vi "OA Get Mode Acq Params.vi"(8 "error in (no error)":errorcluster, 10 "pcListOfParams":string, 11 "pcModeName":string) -> (0 "error out":errorcluster, 2 "pcListOfParams out":string, 3 "function return":u32)   [LabVIEW 2014, in "atmcd32d.lvlib"]
doc: "unsigned int WINAPI OA_GetModeAcqParams(const char * const pcModeName, char * const pcListOfParams);"
uses:
  atmcd32d.lvlib
  atmcd32d.dll
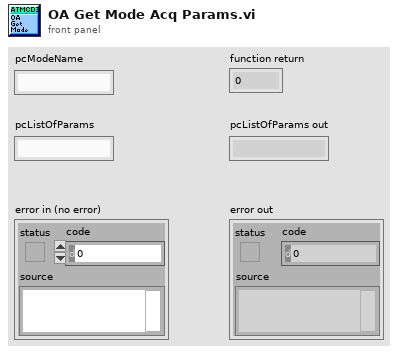
[diagram p1: front panel]
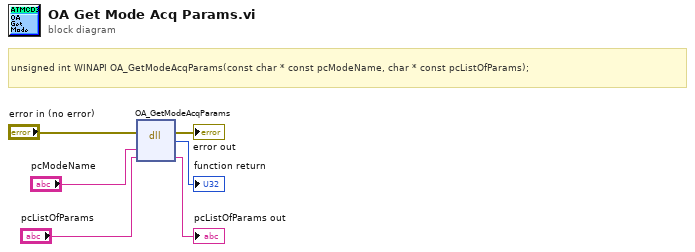
[diagram p0: block diagram]
diagram:
  # "unsigned int WINAPI OA_GetModeAcqParams(const char * const pcModeName, char * const pcListOfParams);"
  n1 = dll-call lib="C:/Users/Bakir/Documents/Lambda2-Testing/lib/Andorlib/atmcd32d.*" fn="OA_GetModeAcqParams"(error in="error in (no error)", "pcModeName"="pcModeName", "pcListOfParams"="pcListOfParams") -> (error out=→"error out":errorcluster, →"function return":u32, "pcListOfParams"=→"pcListOfParams out":string)  [unwired: 3 in, 1 out]
